vi "Nested Aliases.vi"(11 "Self Actor":refnum<class "Self Actor.lvclass">) -> (0 "error out":errorcluster, 2 "Nested Aliases":string[](array[string]))   [LabVIEW 2021, in "jettl.lvlib" / "Self Actor.lvclass"]
uses:
  Self Actor.lvclass
  Self Actor.lvclass/Self Actor.ctl
  jettl.lvlib
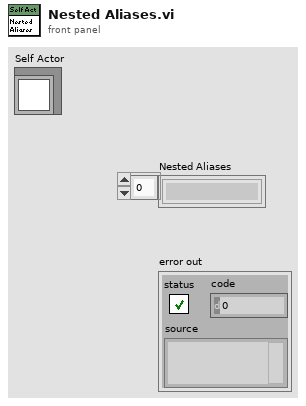
[diagram p1: front panel]
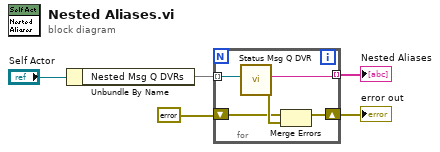
[diagram p0: block diagram]
diagram:
  n1 = Unbundle By Name("Self Actor") -> ("Nested Msg Q DVRs"=w2:set{refnum<data-value>})
  n2 = for {
    tunnel: w2 -> [w10] mode=indexing
    tunnel: [w9] -> w5 mode=indexing
    shift-right: [w7] -> w4
    shift-left: errorcluster {"status"=FALSE, "code"=0, "source"=""} ("error IO") -> [w6]
    n3 = call "Status Msg Q DVR.vi"("Msg Q DVR"=w10) -> ("error out"=w8:errorcluster, "Msg Q DVR Alias"=w9:string)  [unwired: 9 in]
    n4 = Merge Errors(w6, w8) -> (w7:errorcluster)
  }
  "error out" <- w4
  "Nested Aliases" <- w5
